vi "Check for valid Readings.vi"(5 "Min V":dbl, 6 "Init":bool, 7 "Min I":dbl, 8 "PF In":dbl, 9 "VOLTS":dbl, 11 "Current":dbl) -> (0 "PF Out":dbl, 1 "V Out":dbl, 3 "I Out":dbl)   [LabVIEW 2017]
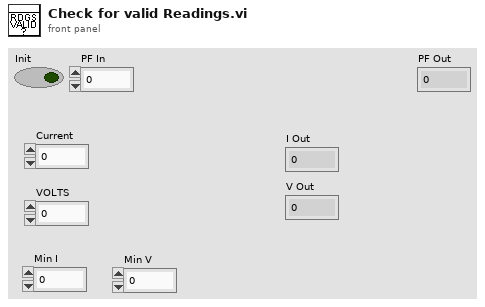
[diagram p1: front panel]
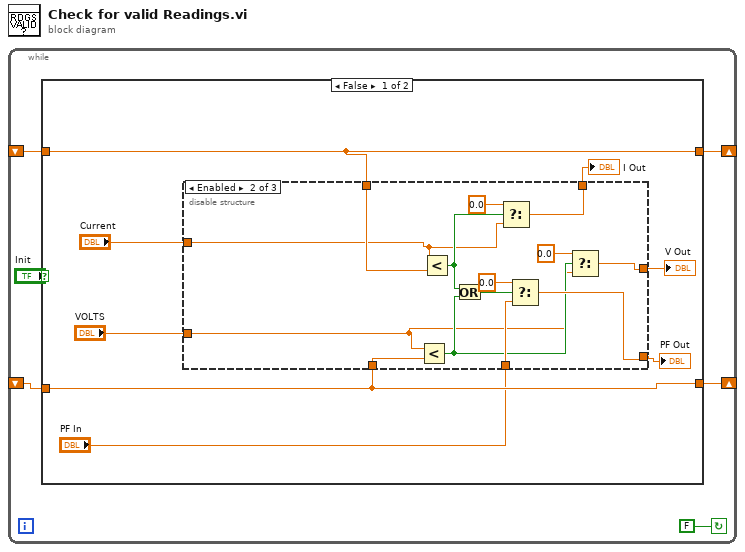
[diagram p0: block diagram]
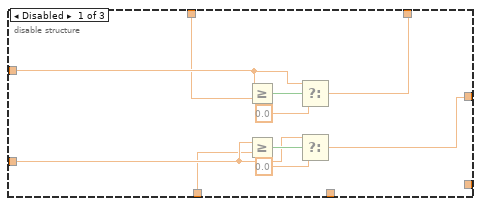
[diagram p2: hidden frame]
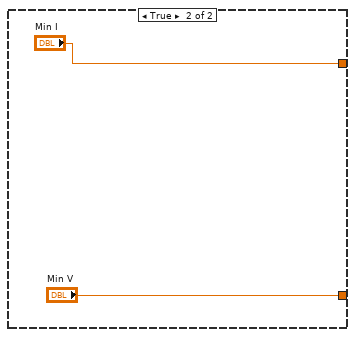
[diagram p4: hidden frame]
diagram:
  n1 = while {
    shift-right: [w3] -> _
    shift-left: _ -> [w2]
    shift-right: [w4] -> _
    shift-left: _ -> [w1]
    stop <- FALSE continue-if-true
    n2 = case shown="False" "Init" {
      tunnel: [w11 "Min V"] -> w4
      tunnel: [w12 "Min I"] -> w3
      tunnel: w2 -> [w12 _]
      tunnel: w1 -> [w11 _]
      frame False {
        n3 = disable-structure shown="Enabled" {
          disable-tunnel: "Current" -> [w20 w30 _]
          disable-tunnel: "VOLTS" -> [w19 w26 _]
          disable-tunnel: w12 -> [w18 w38 _]
          disable-tunnel: w11 -> [w17 w37 _]
          disable-tunnel: [w16 w29 _] -> w10
          disable-tunnel: [w15 w25 _] -> w9
          disable-tunnel: "PF In" -> [_ w35 _]
          disable-tunnel: [_ w34 _] -> w7
          frame Disabled {
            n4 = Greater Or Equal?(x=w20, y=w18) -> (x >= y?=w21:bool)
            n5 = Greater Or Equal?(x=w19, y=w17) -> (x >= y?=w24:bool)
            n6 = Select(t=w20, s=w21, f=0.0) -> (s? t:f=w16:dbl)
            n7 = Select(t=w19, s=w24, f=0.0) -> (s? t:f=w15:dbl)
          }
          frame Enabled {
            n8 = Less?(x=w26, y=w37) -> (x < y?=w28:bool)
            n9 = Less?(x=w30, y=w38) -> (x < y?=w32:bool)
            n10 = Or(x=w32, y=w28) -> (x .or. y?=w36:bool)
            n11 = Select(t=0.0, s=w32, f=w30) -> (s? t:f=w29:dbl)
            n12 = Select(t=0.0, s=w36, f=w35) -> (s? t:f=w34:dbl)
            n13 = Select(t=0.0, s=w28, f=w26) -> (s? t:f=w25:dbl)
          }
          frame Disabled {
          }
        }
        "I Out" <- w10
        "V Out" <- w9
        "PF Out" <- w7
      }
      frame True {
      }
    }
  }
